vi "Dock Instrument.vi"(8 "error in":errorcluster, 10 "Dock":bool, 11 "Instruments in":refnum<class "Instruments.lvclass">) -> (0 "error out":errorcluster, 3 "Instruments out":refnum<class "Instruments.lvclass">)   [LabVIEW 2019]
uses:
  PPL/Subpanel.lvlibp/Subpanel.lvclass
  Library/Instruments.lvclass
  C:/Users/Public/Documents/Development/PPL/Actor Framework.lvlibp/1abvi3w/vi.lib/ActorFramework/Actor/Actor.lvclass
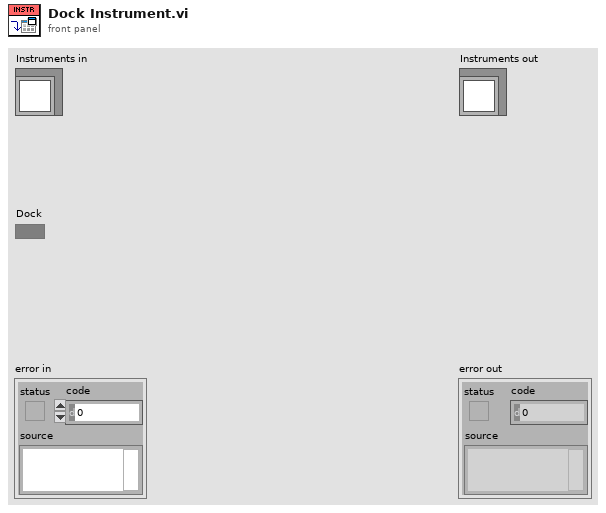
[diagram p1: front panel]
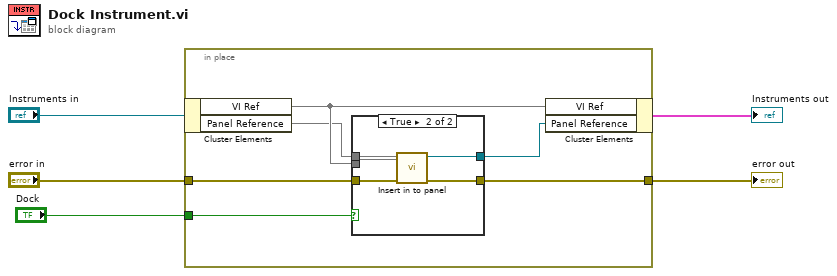
[diagram p0: block diagram]
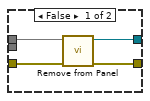
[diagram p2: hidden frame]
diagram:
  n1 = in-place {
    in-place-border: [w10] -> w3
    in-place-border: "error in" -> [w9]
    in-place-border: "Dock" -> [w6]
    n2 = in-place-cluster #1("Instruments in") -> ("VI Ref"=w11, "Panel Reference"=w8)
    n3 = case shown="True" w6 {
      tunnel: w11 -> [_ w20]
      tunnel: [w15 w19] -> w10
      tunnel: w9 -> [w13 w18]
      tunnel: w8 -> [w14 w17]
      tunnel: [w12 w16] -> w7
      frame False {
        n4 = call "Remove from Panel.vi"("error in"=w13, "Subpanel in"=w14) -> ("error out"=w15:errorcluster, "Subpanel out"=w12:refnum<class "Subpanel.lvclass">)  [unwired: 8 in]
      }
      frame True {
        n5 = call "Insert in to panel.vi"("error in"=w18, "VI Ref"=w20, "Subpanel in"=w17) -> ("error out"=w19:errorcluster, "Subpanel out"=w16:refnum<class "Subpanel.lvclass">)  [unwired: 7 in]
      }
    }
    n6 = in-place-cluster #1("VI Ref"=w11, "Panel Reference"=w7) -> (→"Instruments out":cluster{})
  }
  "error out" <- w3
